vi "Komm_Lambdamodul.vi"() -> (0 "A/F":sgl, 1 "O2":sgl, 2 "Ri":sgl, 3 "Lambda":sgl)   [LabVIEW 2020, in "Lambda_ Komm.lvlib"]
uses:
  Lambda_ Komm.lvlib
  Aktion_Lambda.ctl
  FGV Status Lambda Aktionen.ctl
  <vilib>/Instr/_visa.llb/VISA Configure Serial Port (Instr).vi
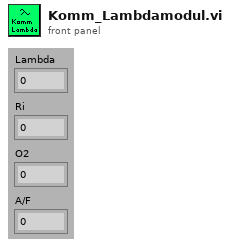
[diagram p1: front panel]
types:
  T1 = typedef "Lambda_ Komm.lvlib/Aktion_Lambda.ctl" = enum16{"Initialisieren", "Kommunikation", "beenden"}
  T2 = typedef "Lambda_ Komm.lvlib/FGV Status Lambda Aktionen.ctl" = enum16{"lesen", "init", "Istwerte"}
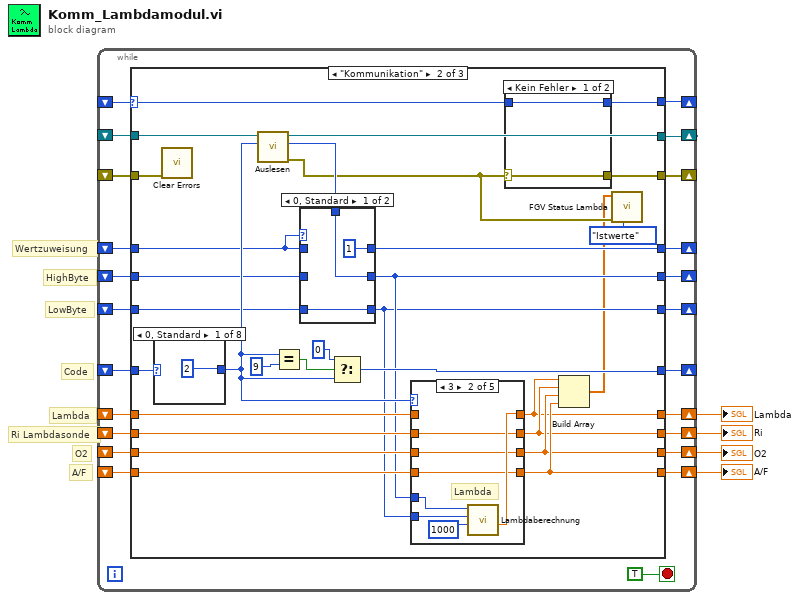
[diagram p0: block diagram]
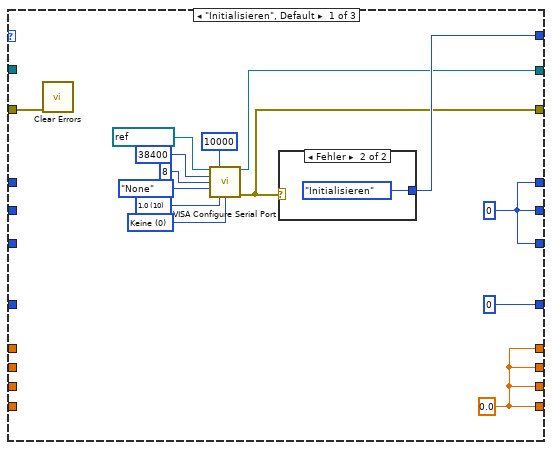
[diagram p2: hidden frame]
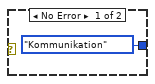
[diagram p3: hidden frame]
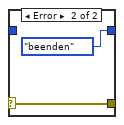
[diagram p4: hidden frame]
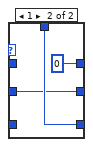
[diagram p5: hidden frame]
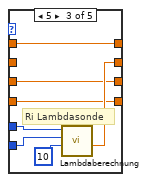
[diagram p7: hidden frame]
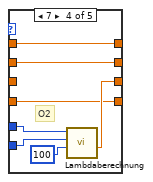
[diagram p8: hidden frame]
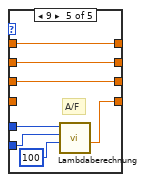
[diagram p9: hidden frame]
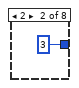
[diagram p10: hidden frame]
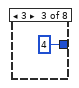
[diagram p11: hidden frame]
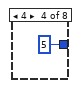
[diagram p12: hidden frame]
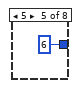
[diagram p13: hidden frame]
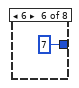
[diagram p14: hidden frame]
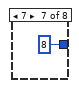
[diagram p15: hidden frame]
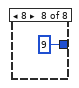
[diagram p16: hidden frame]
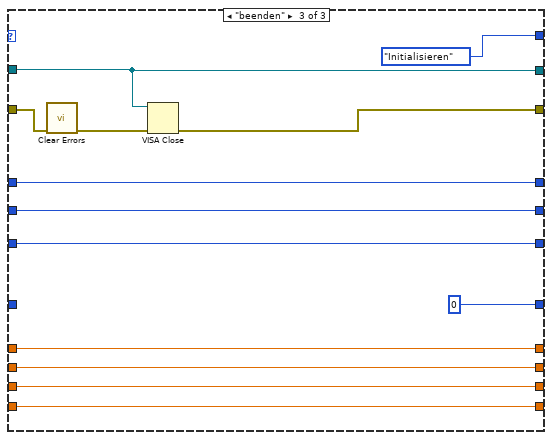
[diagram p17: hidden frame]
diagram:
  # "A/F"
  # "O2"
  # "Ri Lambdasonde"
  # "Lambda"
  # "Wertzuweisung"
  # "Code"
  # "LowByte"
  # "HighByte"
  n1 = while {
    shift-right: [w26] -> _
    shift-left: _ -> [w25]
    shift-right: [w24] -> _
    shift-left: _ -> [w23]
    shift-right: [w21] -> _
    shift-left: _ -> [w22]
    shift-right: [w20] -> _
    shift-left: _ -> [w19]
    shift-right: [w17] -> _
    shift-left: _ -> [w18]
    shift-right: [w14] -> _
    shift-left: _ -> [w16]
    shift-right: [w13] -> _
    shift-left: _ -> [w15]
    shift-right: [w12] -> w4
    shift-left: _ -> [w8]
    shift-right: [w11] -> w3
    shift-left: _ -> [w7]
    shift-right: [w10] -> w2
    shift-left: _ -> [w6]
    shift-right: [w9] -> w1
    shift-left: _ -> [w5]
    stop <- TRUE stop-if-true
    n2 = case shown="\"Kommunikation\"" w25 {
      selector: w25 -> [_ w54 _]
      tunnel: [w41 w53 Aktion_Lambda."Initialisieren" ("Aktion")] -> w26
      tunnel: [w39 w72 w135] -> w24
      tunnel: w23 -> [_ w73 w135]
      tunnel: w22 -> [w28 w44 w126]
      tunnel: [w38 w55 w124] -> w21
      tunnel: [u8 0 ("t") w70 u8 0 ("t")] -> w20
      tunnel: w19 -> [_ w71 _]
      tunnel: w18 -> [_ w65 w133]
      tunnel: [w36 w64 w133] -> w17
      tunnel: w16 -> [_ w62 w132]
      tunnel: w15 -> [_ w61 w131]
      tunnel: [w36 w56 w132] -> w14
      tunnel: [w36 w52 w131] -> w13
      tunnel: [w35 w48 w130] -> w12
      tunnel: [w35 w49 w129] -> w11
      tunnel: [w35 w50 w128] -> w10
      tunnel: [w35 w51 w127] -> w9
      tunnel: w8 -> [_ w60 w130]
      tunnel: w7 -> [_ w59 w129]
      tunnel: w6 -> [_ w58 w128]
      tunnel: w5 -> [_ w57 w127]
      frame "Initialisieren", Default {
        w29 = u16 0 items=["Keine", "XON/XOFF", "RTS/CTS", "XON/XOFF & RTS/CTS", "DTR/DSR", "XON/XOFF & DTR/DSR"] ("flow control (0:none)")
        w30 = u16 10 items=["1.0"=10, "1.5"=15, "2.0"=20] ("stop bits (10: 1 bit)")
        w35 = sgl 0.0 ("Wert")
        w36 = u8 0
        n3 = call <vilib>:"Clear Errors.vi"("error in (no error)"=w28) -> ()  [unwired: 5 in, 2 out]
        n4 = call-poly "VISA Configure Serial Port"("VISA resource name"=refnum<visa-resource-name> "COM3", "timeout (10sec)"=u32 10000, "baud rate (9600)"=u32 38400, "data bits (8)"=u16 8, "parity (0:none)"=enum16{"None", "Odd", "Even", "Mark", "Space"}."None", "stop bits (10: 1 bit)"=w30, "flow control (0:none)"=w29) -> ("VISA resource name out"=w39:refnum<visa-resource-name>, "error out"=w38:errorcluster)  [unwired: 7 in]
        n5 = case shown="Fehler" w38 {
          tunnel: [Aktion_Lambda."Kommunikation" ("Aktion") Aktion_Lambda."Initialisieren" ("Aktion")] -> w41
          frame No Error {
          }
          frame Error {
          }
        }
      }
      frame "Kommunikation" {
        n6 = case shown="0, Standard" w71 {
          tunnel: [u8 2 u8 3 u8 4 u8 5 u8 6 u8 7 u8 8 u8 9] -> w66
          frame 0, Default {
          }
          frame 2 {
          }
          frame 3 {
          }
          frame 4 {
          }
          frame 5 {
          }
          frame 6 {
          }
          frame 7 {
          }
          frame 8 {
          }
        }
        n7 = call <vilib>:"Clear Errors.vi"("error in (no error)"=w44) -> ()  [unwired: 5 in, 2 out]
        n8 = call "Auslesen.vi"("Code"=w66, "VISA-Ressourcenname"=w73) -> ("Fehler (Ausgang)"=w46:errorcluster, "Wert"=w63:u8, "VISA-Ressourcenname (Ausgang)"=w72:refnum<visa-resource-name>)  [unwired: 7 in]
        n9 = Equal?(x=w66, y=u8 9) -> (x = y?=w68:bool)
        n10 = case shown="0, Standard" w65 {
          tunnel: w65 -> [_ _]
          tunnel: [u8 1 u8 0] -> w64
          tunnel: w63 -> [w79 w82]
          tunnel: w62 -> [_ w81]
          tunnel: w61 -> [w78 _]
          tunnel: [w79 w81] -> w56
          tunnel: [w78 w82] -> w52
          frame 0, Default {
          }
          frame 1 {
          }
        }
        n11 = Select(t=u8 0, s=w68, f=w66) -> (s? t:f=w70:u8)
        n12 = case shown="3" w66 {
          tunnel: [w87 w94 w100 w105 w114] -> w48
          tunnel: [w86 w93 w101 w106 w113] -> w49
          tunnel: [w85 w92 w99 w108 w112] -> w50
          tunnel: [w84 w91 w98 w107 w115] -> w51
          tunnel: w60 -> [w87 _ w100 w105 w114]
          tunnel: w59 -> [w86 w93 _ w106 w113]
          tunnel: w58 -> [w85 w92 w99 _ w112]
          tunnel: w57 -> [w84 w91 w98 w107 _]
          tunnel: w56 -> [_ w90 w97 w104 w111]
          tunnel: w52 -> [_ w89 w96 w103 w110]
          frame 0, Default {
          }
          frame 3 {
            # "Lambda"
            n13 = call "Lambdaberechnung.vi"("Nenner"=u16 1000, "LowByte"=w89, "HighByte"=w90) -> ("Wert"=w94:sgl)  [unwired: 8 in]
          }
          frame 5 {
            # "Ri Lambdasonde"
            n14 = call "Lambdaberechnung.vi"("Nenner"=u16 10, "LowByte"=w96, "HighByte"=w97) -> ("Wert"=w101:sgl)  [unwired: 8 in]
          }
          frame 7 {
            # "O2"
            n15 = call "Lambdaberechnung.vi"("Nenner"=u16 100, "LowByte"=w103, "HighByte"=w104) -> ("Wert"=w108:sgl)  [unwired: 8 in]
          }
          frame 9 {
            # "A/F"
            n16 = call "Lambdaberechnung.vi"("Nenner"=u16 100, "LowByte"=w110, "HighByte"=w111) -> ("Wert"=w115:sgl)  [unwired: 8 in]
          }
        }
        n17 = case shown="Kein Fehler" w46 {
          selector: w46 -> [w75 w77]
          tunnel: [w75 w77] -> w55
          tunnel: w54 -> [w74 _]
          tunnel: [w74 Aktion_Lambda."beenden" ("Aktion")] -> w53
          frame No Error {
          }
          frame Error {
          }
        }
        n18 = Build Array(w48, w49, w50, w51) -> (w45:sgl[])
        n19 = call "FGV Status Lambda.vi"("Aktionen"=FGV_Status_Lambda_Aktionen."Istwerte", "error in"=w46, "Istwerte"=w45) -> ()  [unwired: 7 in, 2 out]
      }
      frame "beenden" {
        n20 = call <vilib>:"Clear Errors.vi"("error in (no error)"=w126) -> ("error out"=w125:errorcluster)  [unwired: 5 in, 1 out]
        n21 = VISA Close(VISA resource name=w135, error in (no error)=w125) -> (error out=w124:errorcluster)
      }
    }
  }
  "Lambda" <- w4
  "Ri" <- w3
  "O2" <- w2
  "A/F" <- w1
